vi "Receive Messages.vi"(8 "Error In":errorcluster, 10 "Sender":string, 11 "Communicator in":refnum<class "Communicator.lvclass">) -> (0 "Error Out":errorcluster, 2 "Messages":refnum<class "IMessage.lvclass">[](array[class]), 3 "Communicator out":refnum<class "Communicator.lvclass">)   [LabVIEW 2024, in "Communicator.lvclass"]
uses:
  Communicator.lvclass
  Source/Interfaces/IMessage/IMessage.lvclass
  Source/Interfaces/ICommunicate/ICommunicate.lvclass
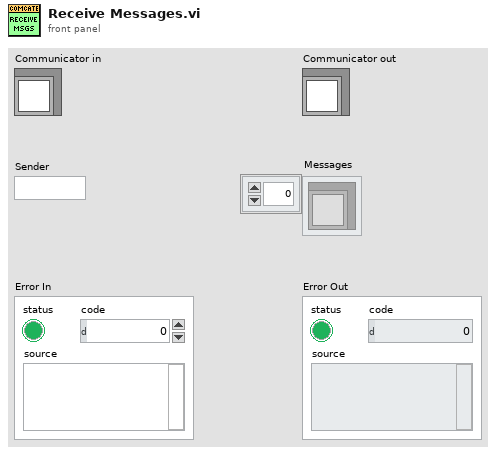
[diagram p1: front panel]
types:
  T1 = typedef "Communicator.lvclass/ObjectAttributes.ctl" = cluster{"IConfigure":refnum<class "IConfigure.lvclass">}
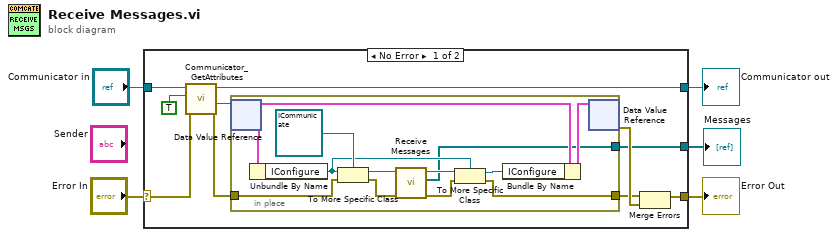
[diagram p0: block diagram]
diagram:
  n1 = case shown="No Error" "Error In" {
    selector: "Error In" -> [w14 w29]
    tunnel: [w11 w29] -> w4
    tunnel: [w12 w28] -> w2
    tunnel: "Communicator in" -> [w15 w28]
    tunnel: [w6 _] -> w1
    frame No Error {
      n2 = call "Communicator_GetAttributes.vi"("Error In"=w14, "OnlyGetDvrReference(False)"=TRUE, "Communicator in"=w15) -> ("Error Out"=w8:errorcluster, "DataRef"=w10:refnum<data-value>, "Communicator out"=w12:refnum<class "Communicator.lvclass">)  [unwired: 5 in, 1 out]
      n3 = in-place {
        in-place-border: w8 -> [w19]
        in-place-border: [w18] -> w7
        in-place-border: [w16] -> w6
        n4 = in-place-dvr #1(w10) -> (w26:T1)  [unwired: 1 out]
        n5 = Unbundle By Name(w26) -> ("IConfigure"=w17:refnum<class "IConfigure.lvclass">)
        n6 = To More Specific Class(target class=refnum<class "ICommunicate.lvclass"> refnum ("ICommunicate.lvclass"), reference=w17, error in=w19) -> (specific class reference=w22:refnum<class "ICommunicate.lvclass">, error out=w23:errorcluster)
        n7 = call-dynamic "Receive Messages.vi"("error in"=w23, "ICommunicate in"=w22) -> ("error out"=w20:errorcluster, "Messages"=w16:refnum<class "IMessage.lvclass">[], "ICommunicate out"=w21:refnum<class "ICommunicate.lvclass">)  [unwired: 7 in]
        n8 = To More Specific Class(target class=w17, reference=w21, error in=w20) -> (specific class reference=w25:refnum<class "IConfigure.lvclass">, error out=w18:errorcluster)
        n9 = Bundle By Name(cluster=w26, "IConfigure"=w25) -> (w27:T1)
        n10 = in-place-dvr #1(w27) -> (w13:errorcluster)  [unwired: 1 out]
      }
      n11 = Merge Errors(w7, w13) -> (w11:errorcluster)
    }
    frame Error {
    }
  }
  "Error Out" <- w4
  "Communicator out" <- w2
  "Messages" <- w1
